vi "Return All Subscriptions.vi"(8 "error in":errorcluster, 11 "NATS Client":refnum<class "NATS Client.lvclass">) -> (0 "error out":errorcluster, 3 "Subscriptions":refnum<class "NATS Subscription.lvclass">[](array[class]))   [LabVIEW 2024, in "NATS Client.lvlib" / "NATS Client.lvclass"]
doc: "Returns all active subscription objects."
uses:
  NATS Client.lvclass
  NATS Subscription/NATS Subscription.lvclass
  NATS Client.lvclass/NATS Client.ctl
  Get subscription map.vi
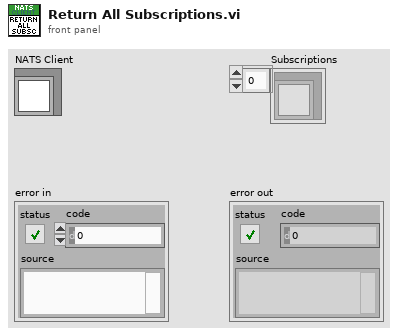
[diagram p1: front panel]
types:
  T1 = typedef "NATS Client.lvlib/NATS Client.lvclass/Subscription Map.ctl" = map{string, refnum<class "NATS Subscription.lvclass">}
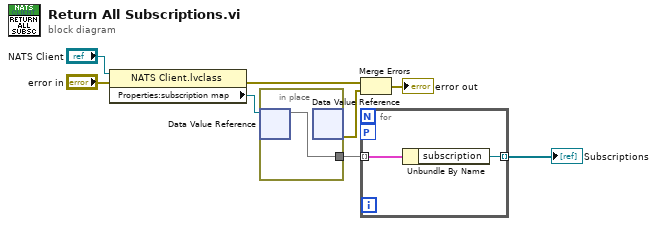
[diagram p0: block diagram]
diagram:
  n1 = property class="NATS Client.lvclass"(reference="NATS Client", error in="error in") -> (error out=w1:errorcluster, "Properties:subscription map"=w7:refnum<data-value>)  [unwired: 1 out]
  n2 = in-place {
    in-place-border: [w9] -> w4
    n3 = in-place-dvr #1(w7) -> (w9:T1)  [unwired: 1 out]
    n4 = in-place-dvr #1() -> (w5:errorcluster)  [unwired: 1 in, 1 out]
  }
  n5 = Merge Errors(w1, w5) -> (→"error out":errorcluster)
  n6 = for {
    tunnel: [w10] -> w3 mode=indexing
    tunnel: w4 -> [w11] mode=indexing
    workers-P: _ -> [_]
    n7 = Unbundle By Name(w11) -> ("subscription"=w10:refnum<class "NATS Subscription.lvclass">)
  }
  "Subscriptions" <- w3
